vi "main.vi"() -> ()   [LabVIEW 2019]
uses:
  <vilib>/silver_ctls/ArrayMatrixCluster/Real Matrix NI_Silver.ctl
  lib/libConvectionDiffusionWrapper/libConvectionDiffusionWrapper.lvlib
panel:
  out "DiffusionValue?":bool
  in  "Stop Button":bool
  in  "Tab Control":enum32{"Control", "Heatmap", "Run Log"}(tab)
  in  "Diffusion Value":dbl=1.0
  in  "Diffusion Switch":enum32{"Value", "Matrix"}(radio)
  in  "Discretization Method":string(combo)="Finite Volumes"
  in  "Source":dbl=1.0
  in  "Reaction Rate":dbl
  in  "Mass Scale":dbl
  in  "Run Button":bool
  in  "Subset":string(combo)="Inner"
  in  "Upwind":string(combo)="Full"
  in  "Grid File":path=path "/home/paul/Schreibtisch/vorlesung-2018/laplace_sample_grid_2d.ugx"
  in  "Solver":string(combo)="Linear Solver"
  in  "Preconditioner":string(combo)="Geometric MultiGrid"
  in  "Max. Iterations":i32=100
  in  "Min. Residuum":dbl=1e-10
  in  "Refinements":i32=3
  in  "Diffusion Matrix Button":bool
  in  "Velocity Vector":dbl[](array[numeric])
  in  "Save As Button":bool
  out "Intensity Graph":dbl[][](graph)
  out "Run Completed":timestamp
  in  "Auto Clear":bool
  in  "Clear Log":bool
  out "Run Log":string
  out "Last Run":timestamp format="%<%x %.3X>T"
  out "Diffusion Matrix":T1
  # "Convection - Diffusion"
  # "Parameter Setup"
  # "Solver Setup"
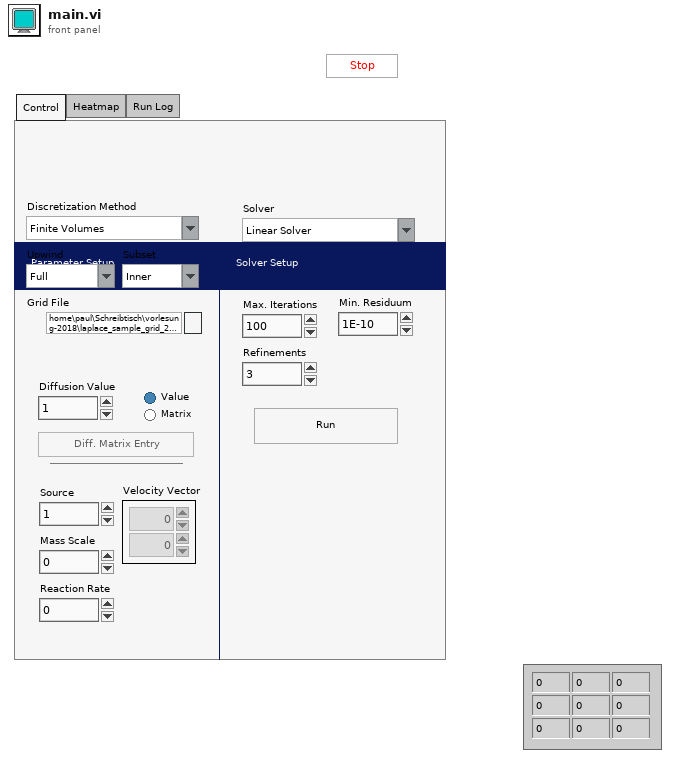
[diagram p1: front panel]
types:
  T1 = typedef "Real Matrix NI_Silver.ctl" = dbl[][]
  T2 = enum8{"Enabled", "Disabled", "Disabled and Grayed Out"}
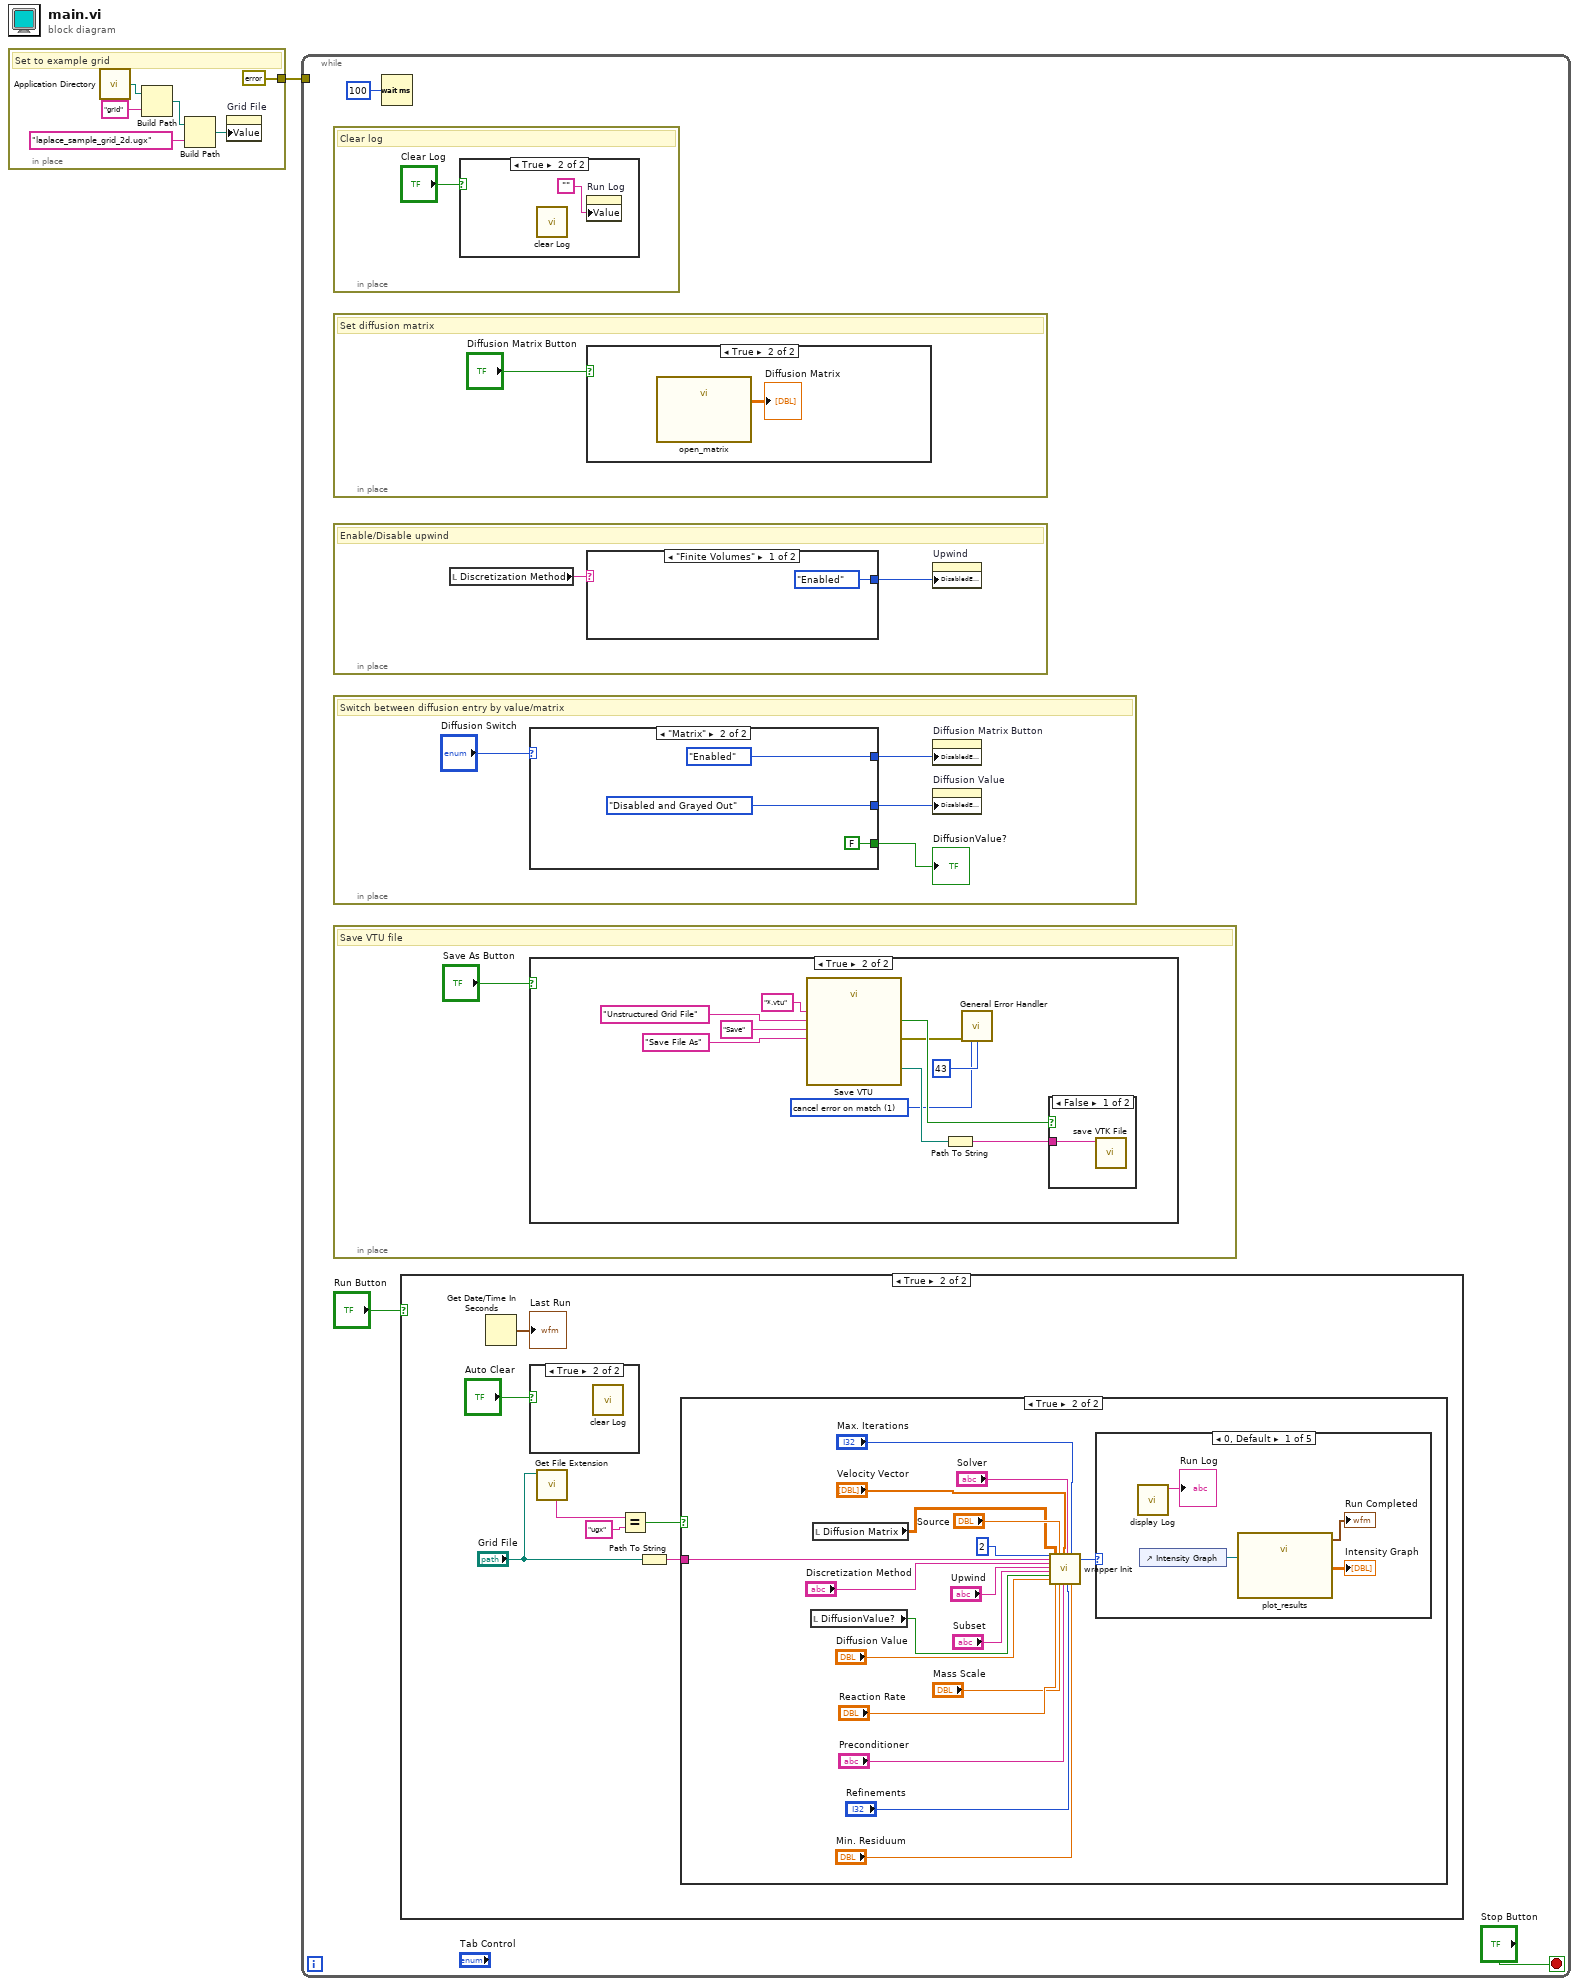
[diagram p0: block diagram]
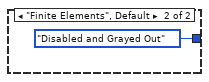
[diagram p2: hidden frame]
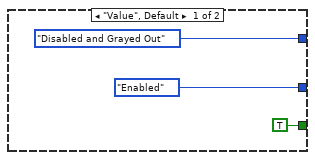
[diagram p5: hidden frame]
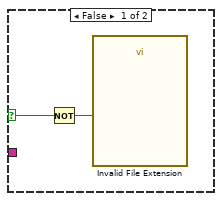
[diagram p10: hidden frame]
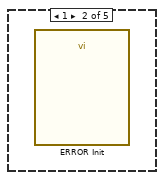
[diagram p11: hidden frame]
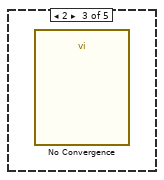
[diagram p12: hidden frame]
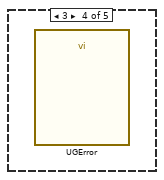
[diagram p13: hidden frame]
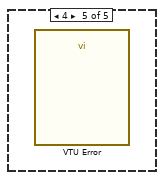
[diagram p14: hidden frame]
diagram:
  n1 = in-place {
    in-place-border: [errorcluster {"status"=FALSE, "code"=0, "source"=""} ("error constant")] -> w1
    # "Set to example grid"
    n2 = call <vilib>:"Application Directory.vi"() -> ("Application Directory"=w7:path)
    n3 = Build Path(base path=w7, name or relative path="grid") -> (appended path=w5:path)
    n4 = Build Path(base path=w5, name or relative path="laplace_sample_grid_2d.ugx") -> (appended path=w3:path)
    n5 = property on="Grid File" class="Path"("Value"=w3) -> ()  [unwired: 2 in, 2 out]
  }
  n6 = while {
    tunnel: w1 -> [_]
    stop <- "Stop Button" stop-if-true
    n7 = in-place {
      # "Clear log"
      n8 = case shown="True" "Clear Log" {
        frame False {
        }
        frame True {
          n9 = call "clear Log.vi"() -> ()  [unwired: 11 in, 1 out]
          n10 = property on="Run Log" class="Str"("Value"="") -> ()  [unwired: 2 in, 2 out]
        }
      }
    }
    n11 = in-place {
      # "Set diffusion matrix"
      n12 = case shown="True" "Diffusion Matrix Button" {
        frame False {
        }
        frame True {
          n13 = call "open_matrix.vi"() -> ("Output Matrix"=→"Diffusion Matrix":T1)  [unwired: 7 in]
        }
      }
    }
    n14 = in-place {
      # "Enable/Disable upwind"
      n15 = local read "Discretization Method"() -> (w12:string)
      n16 = case shown="\"Finite Volumes\"" w12 {
        tunnel: [T2."Enabled" ("Disabled") T2."Disabled and Grayed Out" ("Disabled")] -> w11
        frame "Finite Volumes" {
        }
        frame "Finite Elements", Default {
        }
      }
      n17 = property on="Upwind" class="CmbBox"("DisabledEnum"=w11) -> ()  [unwired: 2 in, 2 out]
    }
    n18 = in-place {
      # "Switch between diffusion entry by value/matrix"
      n19 = case shown="\"Matrix\"" "Diffusion Switch" {
        tunnel: [T2."Enabled" ("Disabled") T2."Disabled and Grayed Out" ("Disabled")] -> w30
        tunnel: [T2."Disabled and Grayed Out" ("Disabled") T2."Enabled" ("Disabled")] -> w29
        tunnel: [TRUE FALSE] -> w27
        frame "Value", Default {
        }
        frame "Matrix" {
        }
      }
      "DiffusionValue?" <- w27
      n20 = property on="Diffusion Matrix Button" class="Bool"("DisabledEnum"=w29) -> ()  [unwired: 2 in, 2 out]
      n21 = property on="Diffusion Value" class="DigNum (strict)"("DisabledEnum"=w30) -> ()  [unwired: 2 in, 2 out]
    }
    n22 = in-place {
      # "Save VTU file"
      n23 = case shown="True" "Save As Button" {
        frame False {
        }
        frame True {
          w16 = 1 items=["no exception", "cancel error on match", "set error on match"] ("[exception action] (none:0)")
          n24 = call "Save VTU"("prompt"="Save File As", "button label"="Save", "pattern (all files)"="*.vtu", "pattern label"="Unstructured Grid File") -> ("selected path"=w20:path, "cancelled"=w21:bool, "error out"=w18:errorcluster)  [unwired: 8 in, 1 out]
          n25 = Path To String(path=w20) -> (string=w19:string)
          n26 = call <vilib>:"General Error Handler.vi"("error in (no error)"=w18, "[exception action] (none:0)"=w16, "[exception code]"=43) -> ()  [unwired: 8 in, 5 out]
          n27 = case shown="False" w21 {
            tunnel: w19 -> [w26 _]
            frame False {
              n28 = call "save VTK File.vi"("path"=w26) -> ()  [unwired: 10 in, 1 out]
            }
            frame True {
            }
          }
        }
      }
    }
    n29 = Wait (ms)(milliseconds to wait=u32 100) -> ()  [unwired: 1 out]
    n30 = case shown="True" "Run Button" {
      frame False {
      }
      frame True {
        n31 = Get Date/Time In Seconds() -> (seconds since 1Jan1904=→"Last Run":timestamp)
        n32 = case shown="True" "Auto Clear" {
          frame False {
          }
          frame True {
            n33 = call "clear Log.vi"() -> ()  [unwired: 11 in, 1 out]
          }
        }
        n34 = call <vilib>:"Get File Extension.vi"("file"="Grid File") -> ("unmodified file extension"=w46:string)  [unwired: 6 in, 4 out]
        n35 = Equal?(x=w46, y="ugx") -> (x = y?=w47:bool)
        n36 = Path To String(path="Grid File") -> (string=w44:string)
        n37 = case shown="True" w47 {
          selector: w47 -> [w48 _]
          tunnel: w44 -> [_ w66]
          frame False {
            n38 = Not(x=w48) -> (.not. x?=w49:bool)
            n39 = call "Invalid File Extension"("Enable"=w49) -> ()  [unwired: 9 in, 2 out]
          }
          frame True {
            n40 = local read "DiffusionValue?"() -> (w65:bool)
            n41 = local read "Diffusion Matrix"() -> (w50:T1)
            n42 = call "wrapper Init.vi"("dim"=2, "fileName"=w66, "discType"="Discretization Method", "upwindType"="Upwind", "subsets"="Subset", "setDiffusionValue"=w65, "diffusionValue"="Diffusion Value", "diffusionMatrix"=w50, "reactionRateValue"="Reaction Rate", "sourceValue"="Source", "massScaleValue"="Mass Scale", "velocityVector"="Velocity Vector", "precondName"="Preconditioner", "solverName"="Solver", "numRefs"="Refinements", "maxNumIter"="Max. Iterations", "absTol"="Min. Residuum") -> ("function return"=w67:i32)  [unwired: 8 in, 2 out]
            n43 = case shown="0, Default" w67 {
              frame 0, Default {
                n44 = call "display Log.vi"() -> ("function return"=→"Run Log":string)  [unwired: 10 in, 1 out]
                n45 = control-ref of="Intensity Graph"() -> (w71:refnum<vi>)
                n46 = call "plot_results.vi"("IntensityGraph in"=w71) -> ("Intensity Graph"=→"Intensity Graph":dbl[][], "Run Completed"=→"Run Completed":timestamp)  [unwired: 9 in]
              }
              frame 1 {
                n47 = call "ERROR Init"() -> ()  [unwired: 10 in, 2 out]
              }
              frame 2 {
                n48 = call "No Convergence"() -> ()  [unwired: 10 in, 2 out]
              }
              frame 3 {
                n49 = call "UGError"() -> ()  [unwired: 10 in, 2 out]
              }
              frame 4 {
                n50 = call "VTU Error"() -> ()  [unwired: 10 in, 2 out]
              }
            }
          }
        }
      }
    }
  }
